vi "stopMotion.vi"(8 "error in (no error)":errorcluster, 10 "model":refnum<class "Model.lvclass">, 11 "ControlledMotionState in":refnum<class "ControlledMotionState.lvclass">) -> (0 "error out":errorcluster, 2 "model 2":refnum<class "Model.lvclass">, 3 "ControlledMotionState out":refnum<class "ControlledMotionState.lvclass">)   [LabVIEW 2013, in "ControlledMotionState.lvclass"]
uses:
  ControlledMotionState.lvclass
  Model/Model/Model.lvclass
  Typedefs/StateSelector.ctl
  EnabledState/EnabledState.lvclass
  Typedefs/M2AADTTypedefs.lvlib
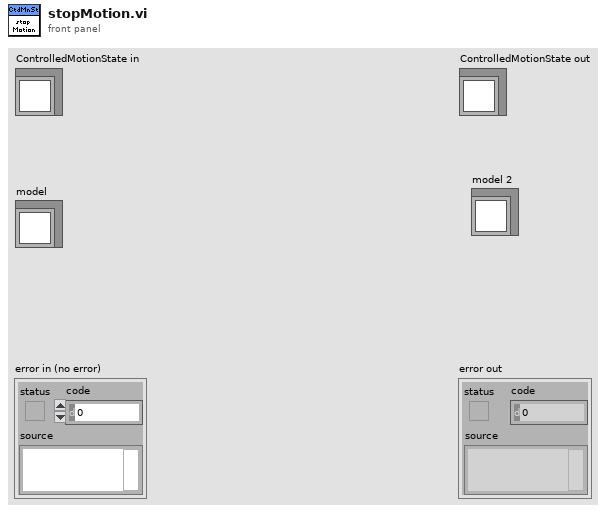
[diagram p1: front panel]
types:
  T1 = typedef "M2AADTTypedefs.lvlib/StateSelector.ctl" = enum16{"EndingCycleState", "FaultState", "InteractiveMotionState", "MovingToNewForceState", "OffState", "PausingState", "StandbyState", "StoppedState"}
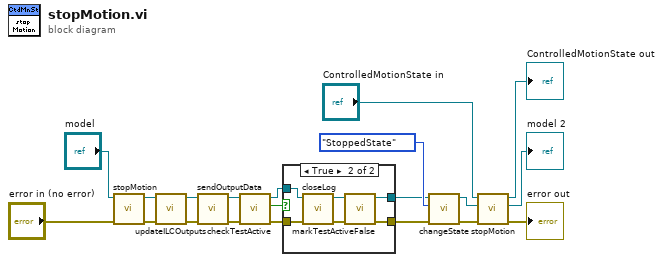
[diagram p0: block diagram]
diagram:
  n1 = call "stopMotion.vi"("error in (no error)"="error in (no error)", "Model in"="model") -> ("error out"=w4:errorcluster, "Model out"=w6:refnum<class "Model.lvclass">)  [unwired: 8 in]
  n2 = call "updateILCOutputs.vi"("error in (no error)"=w4, "Model in"=w6) -> ("error out"=w3:errorcluster, "Model out"=w5:refnum<class "Model.lvclass">)  [unwired: 8 in]
  n3 = call "sendOutputData.vi"("error in (no error)"=w3, "Model in"=w5) -> ("error out"=w1:errorcluster, "Model out"=w2:refnum<class "Model.lvclass">)  [unwired: 8 in]
  n4 = call "checkTestActive.vi"("error in (no error)"=w1, "Model in"=w2) -> ("error out"=w7:errorcluster, "testActiveIsTrue"=w9:bool, "Model out"=w8:refnum<class "Model.lvclass">)  [unwired: 7 in]
  n5 = case shown="True" w9 {
    tunnel: [w22 w25] -> w11
    tunnel: [w21 w23] -> w10
    tunnel: w8 -> [w22 w28]
    tunnel: w7 -> [w21 w27]
    frame False {
    }
    frame True {
      n6 = call "closeLog.vi"("error in (no error)"=w27, "Model in"=w28) -> ("error out"=w24:errorcluster, "Model out"=w26:refnum<class "Model.lvclass">)  [unwired: 8 in]
      n7 = call "markTestActiveFalse.vi"("error in (no error)"=w24, "Model in"=w26) -> ("error out"=w23:errorcluster, "Model out"=w25:refnum<class "Model.lvclass">)  [unwired: 8 in]
    }
  }
  n8 = call "changeState.vi"("error in (no error)"=w10, "State:"=StateSelector."StoppedState", "Model in"=w11) -> ("error out"=w13:errorcluster, "Model out"=w15:refnum<class "Model.lvclass">)  [unwired: 7 in]
  n9 = call-parent "stopMotion.vi"("error in (no error)"=w13, "model"=w15, "State in"="ControlledMotionState in") -> ("error out"=→"error out":errorcluster, "model 2"=→"model 2":refnum<class "Model.lvclass">, "State out"=→"ControlledMotionState out":refnum<class "ControlledMotionState.lvclass">)  [unwired: 6 in]
